vi "Data Generator.vi"(8 "error in":errorcluster, 10 "Initialization Values":T1={"InitializationParams"={"CurrentPartNumber"="a", "MeasurementData"=[{"MeasurementID"=1, "MeasureEnable"=TRUE, "MeasurementPass"=TRUE, "LimitSets"=[{"LimitSetId"=1, "Limits"=[1.5, 2.2]}]}, {"MeasurementID"=2, "MeasureEnable"=TRUE, "MeasurementPass"=TRUE, "LimitSets"=[{"LimitSetId"=1, "Limits"=[1.8, 2.5]}]}, {"MeasurementID"=3, "MeasureEnable"=TRUE, "MeasurementPass"=TRUE, "LimitSets"=[{"LimitSetId"=1, "Limits"=[2.3, 3.2]}]}, {"MeasurementID"=4, "MeasureEnable"=TRUE, "MeasurementPass"=TRUE, "LimitSets"=[{"LimitSetId"=1, "Limits"=[1.6, 2.4]}]}, {"MeasurementID"=5, "MeasureEnable"=TRUE, "MeasurementPass"=TRUE, "LimitSets"=[{"LimitSetId"=1, "Limits"=[2.5, 3.2]}]}]}}, 11 "I":u32) -> (0 "error out":errorcluster, 1 "Defects":bool[](array[boolean]), 2 "Values":dbl[](array[numeric]), 3 "tc":u32, 5 "IsPass":bool=TRUE)   [LabVIEW 2015]
uses:
  <userlib>/_OpenG.lib/numeric/numeric.llb/Random Number Within Range - DBL__ogtk.vi
panel:
  out "l":dbl[](array[numeric])
  out "u":dbl[](array[numeric])
  in  "UCL":dbl[](array[numeric])=[2.3, 2.6, 3.3, 2.5, 3.3]
  in  "LCL":dbl[](array[numeric])=[1.4, 1.7, 2.2, 1.5, 2.4]
types:
  T1 = cluster{"InitializationParams":cluster{"CurrentPartNumber":string, "MeasurementData":cluster{"MeasurementID":i32, "MeasureEnable":bool, "MeasurementPass":bool, "LimitSets":cluster{"LimitSetId":i32, "Limits":dbl[]}[]}[]}}
  T2 = cluster{"MeasurementID":i32, "MeasureEnable":bool, "MeasurementPass":bool, "LimitSets":cluster{"LimitSetId":i32, "Limits":dbl[]}[]}[]
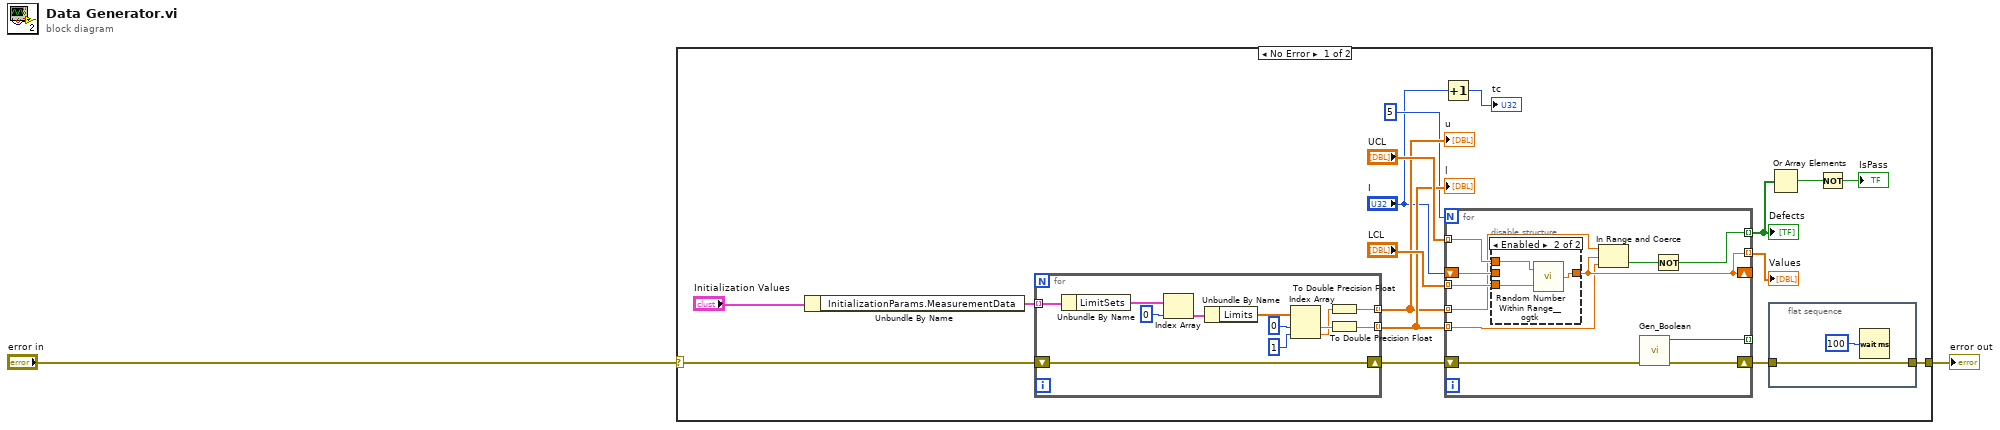
[diagram p0: block diagram]
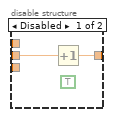
[diagram p2: hidden frame]
diagram:
  n1 = case shown="No Error" "error in" {
    selector: "error in" -> [w5 w50]
    tunnel: [w3 w50] -> w1
    frame No Error {
      n2 = Unbundle By Name("Initialization Values") -> ("InitializationParams.MeasurementData"=w16:T2)
      n3 = for {
        tunnel: w16 -> [w49] mode=indexing
        tunnel: [w40] -> w15 mode=indexing
        tunnel: [w39] -> w14 mode=indexing
        shift-right: [w38] -> w4
        shift-left: w5 -> [w38]
        n4 = Unbundle By Name(w49) -> ("LimitSets"=w46:cluster{"LimitSetId":i32, "Limits":dbl[]}[])
        n5 = Index Array(array=w46, index=0) -> (element=w45:cluster{"LimitSetId":i32, "Limits":dbl[]})
        n6 = Unbundle By Name(w45) -> ("Limits"=w44:dbl[])
        n7 = Index Array(array=w44, index #1=0 ("index"), index #2=1 ("index")) -> (element #1=w42:dbl, element #2=w41:dbl)
        n8 = To Double Precision Float(number=w41) -> (double precision float=w39:dbl)
        n9 = To Double Precision Float(number=w42) -> (double precision float=w40:dbl)
      }
      "u" <- w14
      "l" <- w15
      n10 = Increment(x="I") -> (x+1=→"tc":u32)
      n11 = for {
        N: 5 -> [_]
        shift-right: [w28] -> _
        shift-left: "I" -> [w32]
        tunnel: [w28] -> w9 mode=indexing
        shift-right: [w30] -> w12
        shift-left: w4 -> [w31]
        tunnel: [w29] -> _ mode=indexing
        tunnel: "UCL" -> [w27] mode=indexing
        tunnel: "LCL" -> [w26] mode=indexing
        tunnel: [w22] -> w6 mode=indexing
        tunnel: w15 -> [w24] mode=indexing
        tunnel: w14 -> [w23] mode=indexing
        n12 = disable-structure shown="Enabled" {
          disable-tunnel: w32 -> [w34 _]
          disable-tunnel: [w33 w37] -> w28
          disable-tunnel: w27 -> [_ w36]
          disable-tunnel: w26 -> [_ w35]
          frame Disabled {
            (unwired) TRUE
            n13 = Increment(x=w34) -> (x+1=w33:dbl)
          }
          frame Enabled {
            n14 = call-poly <userlib>:"Random Number Within Range__ogtk.vi"("High"=w36, "Low"=w35) -> ("Random Number"=w37:dbl)  [unwired: 3 in]
          }
        }
        n15 = In Range and Coerce(upper limit=w23, x=w28, lower limit=w24) -> (In Range?=w25:bool)  [unwired: 1 out]
        n16 = call "Gen_Boolean.vi"("error in (no error)"=w31) -> ("error out"=w30:errorcluster, "Boolean"=w29:bool)  [unwired: 9 in]
        n17 = Not(x=w25) -> (.not. x?=w22:bool)
      }
      "Values" <- w9
      "Defects" <- w6
      n18 = flat-sequence {
        tunnel: w12 -> [w21]
        tunnel: [w21] -> w3
        frame #0 {
          n19 = Wait (ms)(milliseconds to wait=u32 100) -> ()  [unwired: 1 out]
        }
      }
      n20 = Or Array Elements(Boolean array=w6) -> (logical OR=w8:bool)
      n21 = Not(x=w8) -> (.not. x?=→"IsPass":bool)
    }
    frame Error {
    }
  }
  "error out" <- w1
